vi "Compress.vi"(0 "instrument handle":refnum<k15>, 1 "Length":dbl, 2 "RepeatLimit":i32 format="%.0g", 5 "Trace":string="Trace1" caption="trace name (Trace1)", 7 "Method (Block)":i32(ring) items=["Block", "Cfit", "Maximum", "Mean", "Minimum", "Sample", "rms", "Deviation"], 9 "StartOffset":dbl, 11 "error in (no error)":errorcluster {"code" format="%.0x"}, 12 "RepeatOffset":dbl, 13 "ValBufferSize":i32=2048 caption="ValBufferSize (2048)") -> (4 "instrument handle out":refnum<k15>, 6 "Val":dbl[](array[numeric]) format="%.2p", 8 "ValActualSize":i32, 15 "error out":errorcluster {"code" format="%.0x"})   [LabVIEW 2009, in "Keysight XSAn.lvlib"]
doc: "Returns compressed data for the specified trace data. The data is returned in the same units as the original trace and only works with the currently selected measurement.\n\nSupported Models: M9290A, N8973B, N8974B, N8975B, N8976B, N9000A, N9000B, N9010A, N9010B, N9020A, N9020B, N9030A, N9030B, N9038A, N9040B, N9041B, SPN9003A, SPN9026A"
uses:
  <instrlib>/Keysight XSAn/Keysight XSAn.lvlib
  AgXSAn.dll
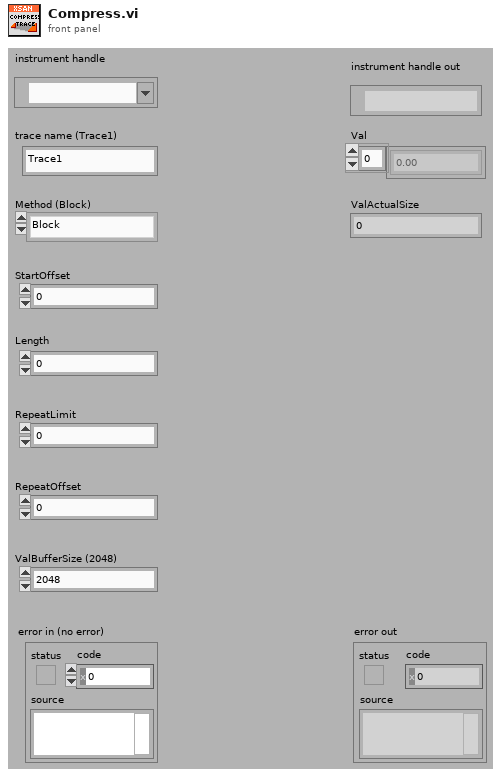
[diagram p1: front panel]
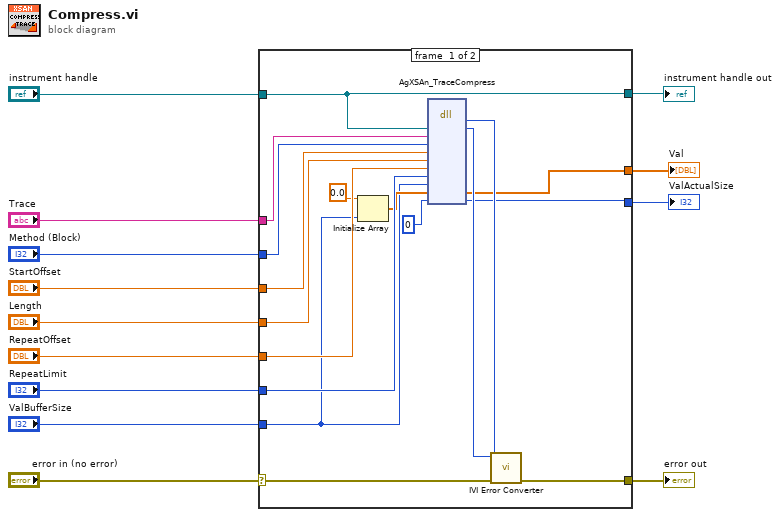
[diagram p0: block diagram]
diagram:
  n1 = case shown="No Error" "error in (no error)" {
    selector: "error in (no error)" -> [w28 w32]
    tunnel: [w27 w32] -> w13
    tunnel: "instrument handle" -> [w15 w31]
    tunnel: "Trace" -> [w26 _]
    tunnel: "Method (Block)" -> [w25 _]
    tunnel: "StartOffset" -> [w24 _]
    tunnel: "Length" -> [w23 _]
    tunnel: "RepeatOffset" -> [w22 _]
    tunnel: "RepeatLimit" -> [w21 _]
    tunnel: "ValBufferSize" -> [w14 _]
    tunnel: [w18 _] -> w3
    tunnel: [w16 _] -> w2
    tunnel: [w15 w31] -> w1
    frame #0 {
      n2 = Initialize Array(0.0 ("element"), w14) -> (w20:dbl[])
      n3 = dll-call lib="AgXSAn**.dll" fn="AgXSAn_TraceCompress"("Vi"=w15, "Trace"=w26, "Method"=w25, "StartOffset"=w24, "Length"=w23, "RepeatOffset"=w22, "RepeatLimit"=w21, "ValBufferSize"=w14, "Val"=w20, "ValActualSize"=0) -> (w29:i32, "Vi"=w30:u32, "Val"=w18:dbl[], "ValActualSize"=w16:i32)  [unwired: 10 in, 2 out]
      n4 = call <instrlib>:"IVI Error Converter.vi"("error in (no error)"=w28, "IVI error code (0)"=w29, "instrument handle"=w30) -> ("error out"=w27:errorcluster)  [unwired: 7 in, 1 out]
    }
    frame #1 {
    }
  }
  "error out" <- w13
  "instrument handle out" <- w1
  "Val" <- w3
  "ValActualSize" <- w2
